vi "Clear Packages.vi"() -> ()   [LabVIEW 2019]
uses:
  Controls/OCR_ClearPackage_ActioParam.ctl
panel:
  in  "OCR_Exit":bool
  in  "OCR_Remove":bool
  in  "Tab Control":enum32{"Trained Package", "Training Example"}(tab)
  in  "Trained Packaged Data":i32(listbox)
  in  "Training Package":i32(listbox)
  in  "Training Example List":i32(listbox)
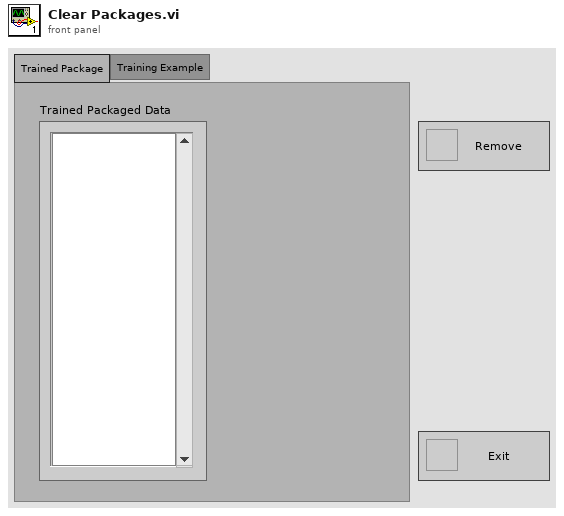
[diagram p1: front panel]
types:
  T1 = typedef "OCR_ClearPackage_ActioParam.ctl" = cluster{"OCR_ClearPackage_Action":enum16{"Init", "UpdateTrainedDataList", "UpdatePackageNumberList", "Remove", "Exit"}, "OCR_ClearPackage_Param":variant}
  T2 = enum16{"Init", "UpdateTrainedDataList", "UpdatePackageNumberList", "Remove", "Exit"}
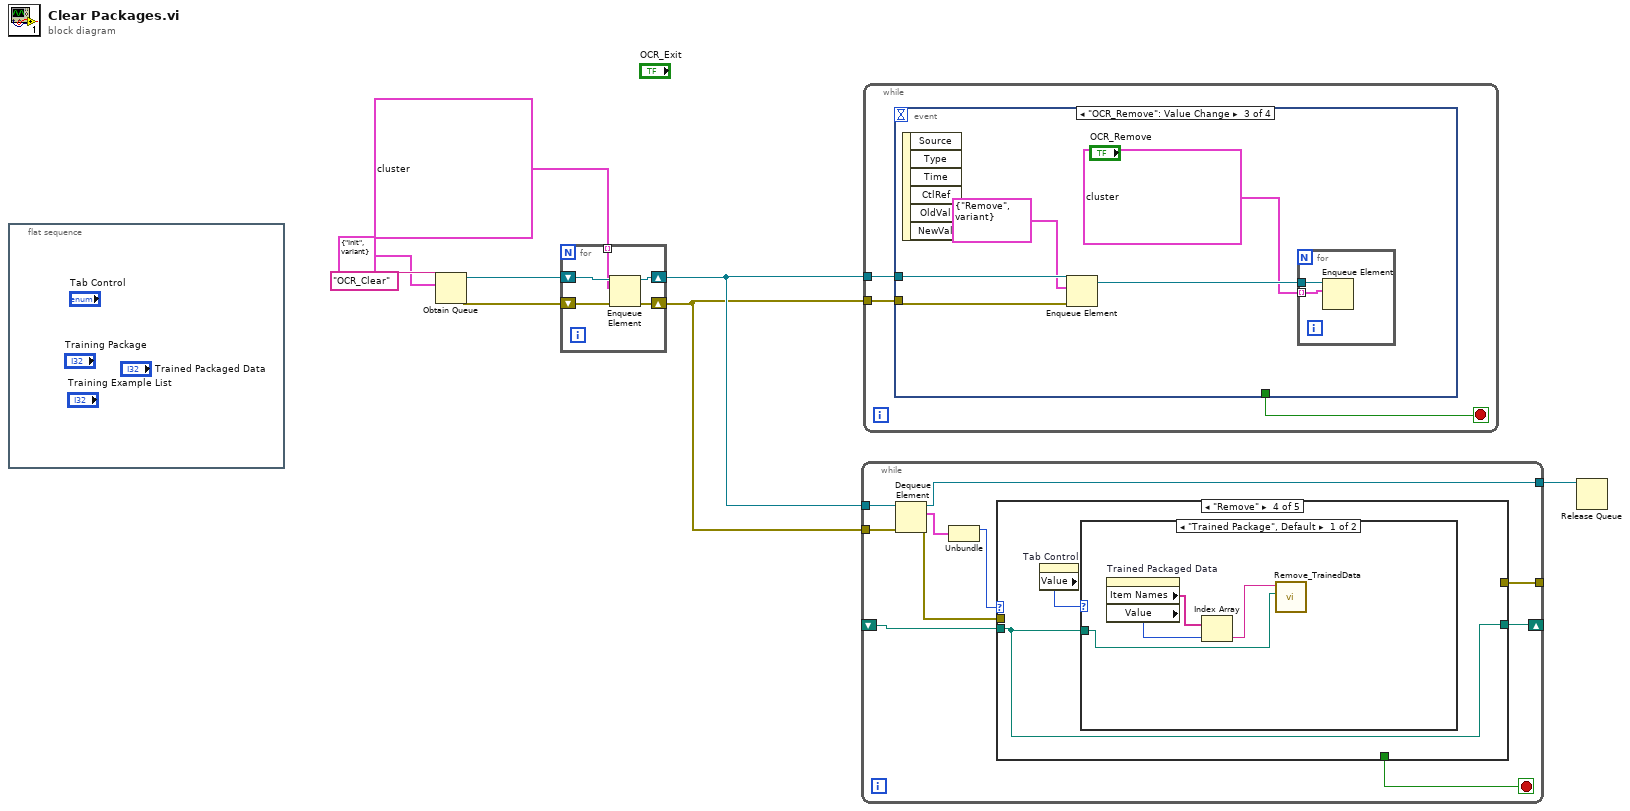
[diagram p0: block diagram]
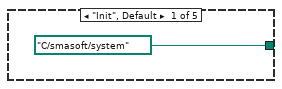
[diagram p2: hidden frame]
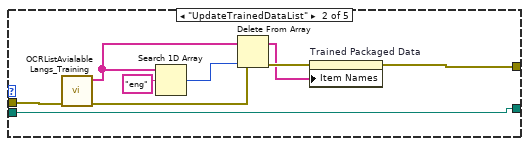
[diagram p3: hidden frame]
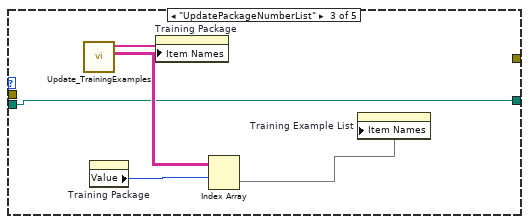
[diagram p4: hidden frame]
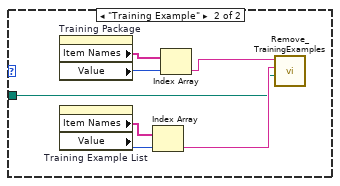
[diagram p5: hidden frame]
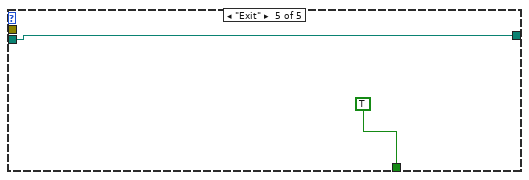
[diagram p6: hidden frame]
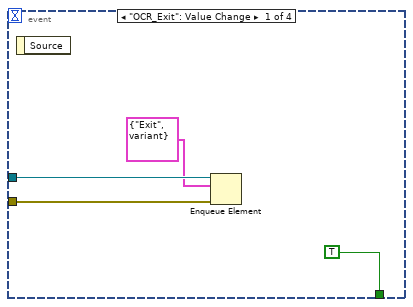
[diagram p7: hidden frame]
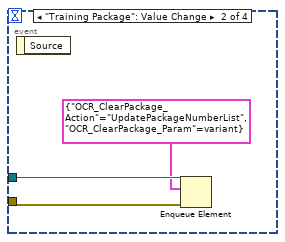
[diagram p8: hidden frame]
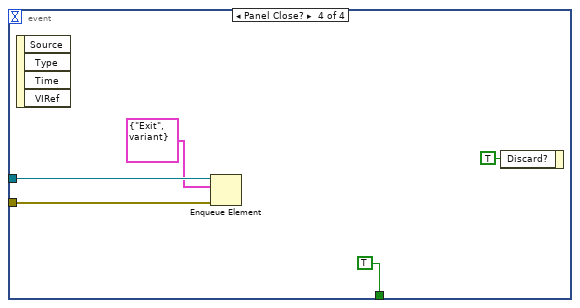
[diagram p9: hidden frame]
diagram:
  n1 = flat-sequence {
    frame #0 {
    }
  }
  n2 = Obtain Queue(name (unnamed)="OCR_Clear", element data type=T1 {"OCR_ClearPackage_Action"=enum."Init", "OCR_ClearPackage_Param"=variant} ("OCR_ClearPackage_ActioParam")) -> (queue out=w5:refnum<queue>, error out=w3:errorcluster)  [unwired: 3 in, 1 out]
  n3 = for {
    tunnel: T1[] [{"OCR_ClearPackage_Action"=enum."Init", "OCR_ClearPackage_Param"=variant}, {"OCR_ClearPackage_Action"=enum."UpdatePackageNumberList", "OCR_ClearPackage_Param"=variant}, {"OCR_ClearPackage_Action"=enum."UpdateTrainedDataList", "OCR_ClearPackage_Param"=variant}] ("element") -> [w9] mode=indexing
    shift-right: [w12] -> w4
    shift-left: w5 -> [w13]
    shift-right: [w10] -> w2
    shift-left: w3 -> [w11]
    n4 = Enqueue Element(queue=w13, element=w9, error in (no error)=w11) -> (queue out=w12:refnum<queue>, error out=w10:errorcluster)  [unwired: 1 in, 1 out]
  }
  n5 = while {
    tunnel: w4 -> [w23]
    tunnel: w2 -> [w22]
    tunnel: [w21] -> w6
    tunnel: [w16] -> _
    shift-right: [w15] -> _
    shift-left: _ -> [w14]
    stop <- w18 stop-if-true
    n6 = Dequeue Element(queue=w23, error in (no error)=w22) -> (queue out=w21:refnum<queue>, element=w20:T1, error out=w17:errorcluster)  [unwired: 1 in, 1 out]
    n7 = Unbundle(w20) -> ("OCR_ClearPackage_Action"=w19:T2)  [unwired: 1 out]
    n8 = case shown="\"Remove\"" w19 {
      tunnel: [_ _ _ _ TRUE ("Discard?")] -> w18
      tunnel: w17 -> [_ w32 _ _ _]
      tunnel: [_ w30 _ _ _] -> w16
      tunnel: [path "C:/smasoft/system" ("rooth path") w29 w33 w38 w51] -> w15
      tunnel: w14 -> [_ w29 w33 w38 w51]
      frame "Init", Default {
      }
      frame "UpdateTrainedDataList" {
        n9 = call "OCRListAvialableLangs_Training.vi"("error in (no error)"=w32) -> ("error out"=w31:errorcluster, "Langs"=w27:string[])  [unwired: 9 in]
        n10 = Search 1D Array(1D array=w27, element="eng") -> (index of element=w26:i32)  [unwired: 1 in]
        n11 = Delete From Array(array=w27, index=w26) -> (array with subset deleted=w25:string[])  [unwired: 1 in, 1 out]
        n12 = property on="Trained Packaged Data" class="LstBox (strict)"(error in=w31, "Item Names"=w25) -> (error out=w30:errorcluster)  [unwired: 1 in, 1 out]
      }
      frame "UpdatePackageNumberList" {
        n13 = call "Update_TrainingExamples.vi"() -> ("training number"=w35:string[][], "package"=w37:string[])  [unwired: 9 in, 1 out]
        n14 = property on="Training Package" class="LstBox (strict)"() -> ("Value"=w36:i32)  [unwired: 2 in, 2 out]
        n15 = property on="Training Package" class="LstBox (strict)"("Item Names"=w37) -> ()  [unwired: 2 in, 2 out]
        n16 = Index Array(array=w35, index (row)=w36) -> (element=w34:string[])  [unwired: 1 in]
        n17 = property on="Training Example List" class="LstBox (strict)"("Item Names"=w34) -> ()  [unwired: 2 in, 2 out]
      }
      frame "Remove" {
        n18 = property on="Tab Control" class="TabCtl (strict)"() -> ("Value"=w39:enum32{"Trained Package", "Training Example"})  [unwired: 2 in, 2 out]
        n19 = case shown="\"Trained Package\", Default" w39 {
          tunnel: w38 -> [w40 w44]
          frame "Trained Package", Default {
            n20 = property on="Trained Packaged Data" class="LstBox (strict)"() -> ("Item Names"=w43:string[], "Value"=w42:i32)  [unwired: 2 in, 2 out]
            n21 = Index Array(array=w43, index=w42) -> (element=w41:string)
            n22 = call "Remove_TrainedData.vi"("File Path Control"=w40, "TrainnedData"=w41) -> ()  [unwired: 10 in]
          }
          frame "Training Example" {
            n23 = property on="Training Package" class="LstBox (strict)"() -> ("Item Names"=w50:string[], "Value"=w49:i32)  [unwired: 2 in, 2 out]
            n24 = property on="Training Example List" class="LstBox (strict)"() -> ("Item Names"=w48:string[], "Value"=w47:i32)  [unwired: 2 in, 2 out]
            n25 = Index Array(array=w48, index=w47) -> (element=w45:string)
            n26 = Index Array(array=w50, index=w49) -> (element=w46:string)
            n27 = call "Remove_TrainingExamples.vi"("rooth path"=w44, "number"=w45, "package"=w46) -> ()  [unwired: 9 in]
          }
        }
      }
      frame "Exit" {
      }
    }
  }
  n28 = while {
    tunnel: w4 -> [w55]
    tunnel: w2 -> [w54]
    stop <- w53 stop-if-true
    n29 = event shown="[2] \"OCR_Remove\": Value Change" {
      selector: _ -> [_ _ _ _]
      dyn-events: _ -> [_ _ _ _]
      timeout: _ -> [_ _ _ _]
      tunnel: w55 -> [w59 w62 w67 w74]
      tunnel: w54 -> [w58 w61 w66 w73]
      tunnel: [TRUE ("Discard?") _ _ TRUE ("Discard?")] -> w53
      event "OCR_Exit": Value Change {
        n30 = event-data() -> ()  [unwired: 1 in, 1 out]
        n31 = Enqueue Element(queue=w59, element=T1 {"OCR_ClearPackage_Action"=enum."Exit", "OCR_ClearPackage_Param"=variant}, error in (no error)=w58) -> ()  [unwired: 1 in, 3 out]
      }
      event "Training Package": Value Change {
        n32 = event-data() -> ()  [unwired: 1 in, 1 out]
        n33 = Enqueue Element(queue=w62, element=T1 {"OCR_ClearPackage_Action"=enum."UpdatePackageNumberList", "OCR_ClearPackage_Param"=variant}, error in (no error)=w61) -> ()  [unwired: 1 in, 3 out]
      }
      event "OCR_Remove": Value Change {
        n34 = event-data() -> ()  [unwired: 1 in, 6 out]
        n35 = Enqueue Element(queue=w67, element=T1 {"OCR_ClearPackage_Action"=enum."Remove", "OCR_ClearPackage_Param"=variant}, error in (no error)=w66) -> (queue out=w64:refnum<queue>)  [unwired: 1 in, 2 out]
        n36 = for {
          tunnel: w64 -> [w69]
          tunnel: T1[] [{"OCR_ClearPackage_Action"=enum."UpdatePackageNumberList", "OCR_ClearPackage_Param"=variant}, {"OCR_ClearPackage_Action"=enum."UpdateTrainedDataList", "OCR_ClearPackage_Param"=variant}] ("element") -> [w68] mode=indexing
          n37 = Enqueue Element(queue=w69, element=w68) -> ()  [unwired: 2 in, 3 out]
        }
      }
      event Panel Close? {
        n38 = event-data() -> ()  [unwired: 1 in, 4 out]
        n39 = Enqueue Element(queue=w74, element=T1 {"OCR_ClearPackage_Action"=enum."Exit", "OCR_ClearPackage_Param"=variant}, error in (no error)=w73) -> ()  [unwired: 1 in, 3 out]
        n40 = event-data("Discard?"=TRUE) -> ()  [unwired: 1 in, 1 out]
      }
    }
  }
  n41 = Release Queue(queue=w6) -> ()  [unwired: 2 in, 3 out]
